vi "ANNN.vi"(11 "Variables and Memory in":T1 {"GFX" format="%02x"}) -> (3 "Variables and Memory out":T1 {"GFX" format="%02x"})   [LabVIEW 2021]
uses:
  Controls/ClusterF.ctl
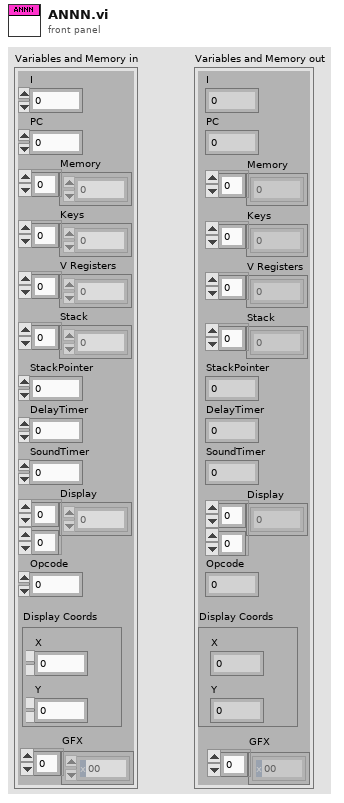
[diagram p1: front panel]
types:
  T1 = typedef "ClusterF.ctl" = cluster{"I":u16, "PC":u16, "Memory":u8[], "Keys":u8[], "V Registers":u8[], "Stack":u16[], "StackPointer":u16, "DelayTimer":u8, "SoundTimer":u8, "Display":u8[][], "Opcode":u16, "Display Coords":cluster{"X":u8, "Y":u8}, "GFX":u8[]}
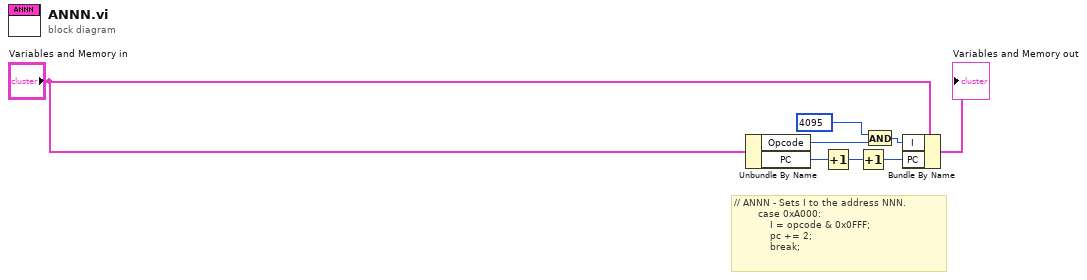
[diagram p0: block diagram]
diagram:
  # "// ANNN - Sets I to the address NNN.\n        case 0xA000:\n            I = opcode & 0x0FFF;\n            pc += 2;\n            break;"
  n1 = Unbundle By Name("Variables and Memory in") -> ("Opcode"=w8:u16, "PC"=w5:u16)
  n2 = Increment(x=w5) -> (x+1=w4:u16)
  n3 = Increment(x=w4) -> (x+1=w6:u16)
  n4 = And(x=u16 4095 ("y"), y=w8) -> (x .and. y?=w3:u16)
  n5 = Bundle By Name(cluster="Variables and Memory in", "I"=w3, "PC"=w6) -> (→"Variables and Memory out":T1)
